vi "Stop Core.vi"(10 "final error code":i32, 11 "Async Actor Example in":refnum<class "Async Methods Actor Example.lvclass">) -> (3 "Async Actor Example out":refnum<class "Async Methods Actor Example.lvclass">)   [LabVIEW 2021, in "Async Methods Actor Example.lvlib" / "Async Methods Actor Example.lvclass"]
doc: "(<B>Filename</B>: Actor Framework.lvlib:Actor.lvclass:Stop Core.vi)\n\nDefines what the actor does before it stops. Use the <B>final error code</B> input to determine whether the actor shut down in response to an error.\n\nBy default, this method passes the Stop message along to all auto-stop nested actors. A descendant class may override this method to define additional behavior, such as shutting down any processes the actor initiated in its override of the Actor Core method."
uses:
  Async Methods Actor Example.lvclass
  Async Methods Actor Example.lvclass/Async Methods Actor Example.ctl
  Async Methods Actor/Async Methods Actor/Async Methods Actor.lvclass
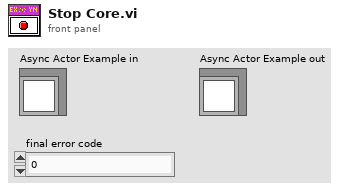
[diagram p1: front panel]
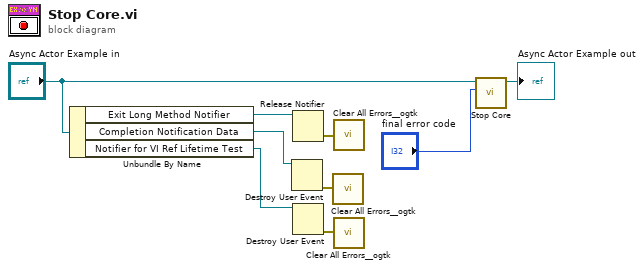
[diagram p0: block diagram]
diagram:
  n1 = Unbundle By Name("Async Actor Example in") -> ("Exit Long Method Notifier"=w6:refnum<notifier>, "Completion Notification Data"=w4:refnum<user-event>, "Notifier for VI Ref Lifetime Test"=w1:refnum<user-event>)
  n2 = Destroy User Event(user event=w4) -> (error out=w3:errorcluster)  [unwired: 1 in]
  n3 = Release Notifier(notifier=w6) -> (error out=w5:errorcluster)  [unwired: 2 in, 2 out]
  n4 = Destroy User Event(user event=w1) -> (error out=w2:errorcluster)  [unwired: 1 in]
  n5 = call <userlib>:"Clear All Errors__ogtk.vi"("Error In"=w3) -> ()  [unwired: 3 in, 1 out]
  n6 = call <userlib>:"Clear All Errors__ogtk.vi"("Error In"=w5) -> ()  [unwired: 3 in, 1 out]
  n7 = call <userlib>:"Clear All Errors__ogtk.vi"("Error In"=w2) -> ()  [unwired: 3 in, 1 out]
  n8 = call-parent "Stop Core.vi"("final error code"="final error code", "Async Methods Actor in"="Async Actor Example in") -> ("Async Methods Actor out"=→"Async Actor Example out":refnum<class "Async Methods Actor Example.lvclass">)  [unwired: 9 in]
